vi "Potential Divider Calc.vi"() -> ()   [LabVIEW 2013]
panel:
  in  "Vout":dbl(slide) scale=0.0..24.0
  in  "Rb":dbl(slide) scale=0.0..10.0
  in  "Ra":dbl(slide) scale=0.0..10.0
  in  "Vin":dbl(slide) scale=0.0..24.0
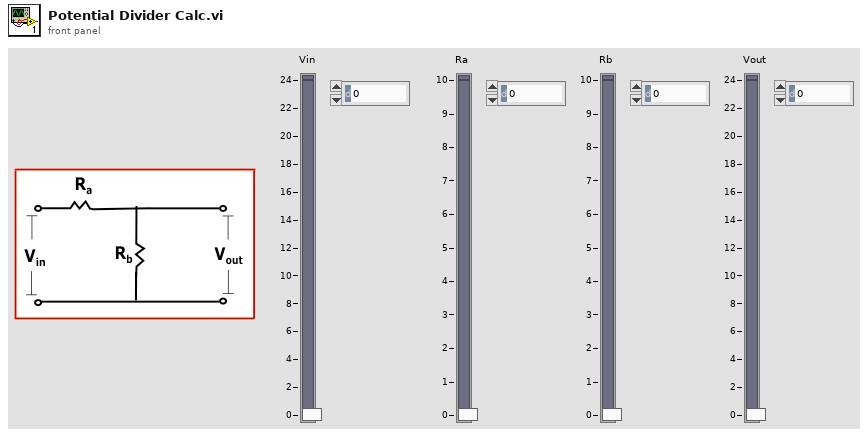
[diagram p1: front panel]
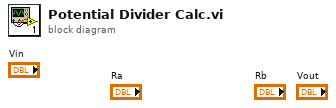
[diagram p0: block diagram]
diagram:
